vi "GetProperties.vi"(8 "error in":errorcluster, 11 "Boolean in":refnum<class "Boolean.lvclass">) -> (0 "error out":errorcluster, 3 "Boolean out":refnum<class "Boolean.lvclass">)   [LabVIEW 2014, in "Boolean.lvclass"]
uses:
  Boolean.lvclass
  Boolean.lvclass/Boolean.ctl
  Control/Control.lvclass
  Text/Text.lvclass
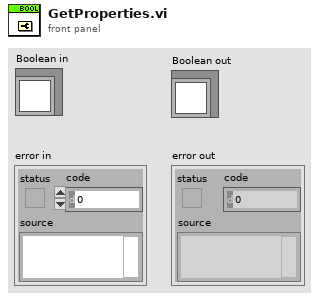
[diagram p1: front panel]
types:
  T1 = typedef "LVBoundsTypeDef.ctl" = cluster{"Width":u32, "Height":u32}
  T2 = typedef "LVKeyTypeDef.ctl" = cluster{"Focus":bool, "Control":bool, "Shift":bool, "Key":string}
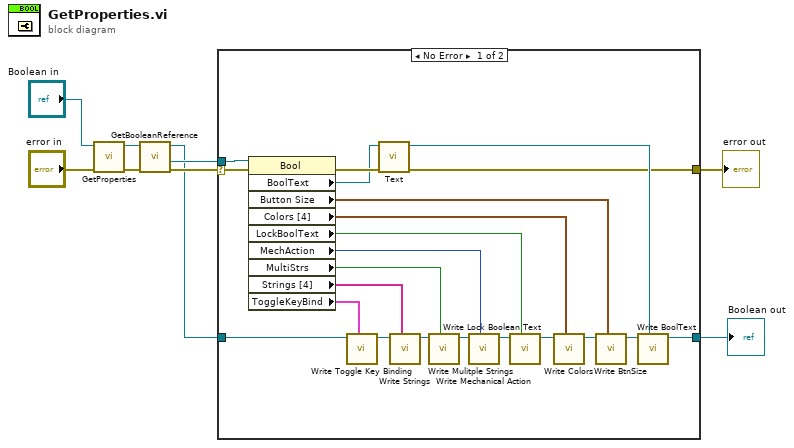
[diagram p0: block diagram]
diagram:
  n1 = call-parent "GetProperties.vi"("error in"="error in", "Control in"="Boolean in") -> ("error out"=w6:errorcluster, "Control out"=w7:refnum<class "Boolean.lvclass">)  [unwired: 8 in]
  n2 = call "GetBooleanReference.vi"("error in"=w6, "Boolean in"=w7) -> ("error out"=w5:errorcluster, "Boolean reference"=w4:refnum<vi>, "Boolean out"=w3:refnum<class "Boolean.lvclass">)  [unwired: 7 in]
  n3 = case shown="No Error" w5 {
    selector: w5 -> [w31 w32]
    tunnel: w4 -> [w30 _]
    tunnel: w3 -> [w12 w33]
    tunnel: [w11 w33] -> w1
    tunnel: [w10 w32] -> w2
    frame No Error {
      n4 = property class="Bool"(reference=w30, error in=w31) -> (error out=w29:errorcluster, "BoolText"=w28:refnum<vi>, "Button Size"=w24:T1, "Colors [4]"=w23:cluster{u32, u32}[], "LockBoolText"=w22:bool, "MechAction"=w19:u32, "MultiStrs"=w17:bool, "Strings [4]"=w15:string[], "ToggleKeyBind"=w13:T2)  [unwired: 1 out]
      n5 = call "Write Toggle Key Binding.vi"("Toggle Key Binding"=w13, "Boolean in"=w12) -> ("Boolean out"=w14:refnum<class "Boolean.lvclass">)  [unwired: 7 in]
      n6 = call "Text.vi"("error in"=w29, "GObj Refnum"=w28) -> ("error out"=w10:errorcluster, "Text out"=w25:refnum<class "Text.lvclass">)  [unwired: 8 in]
      n7 = call "Write Strings.vi"("Strings"=w15, "Boolean in"=w14) -> ("Boolean out"=w16:refnum<class "Boolean.lvclass">)  [unwired: 7 in]
      n8 = call "Write Mulitple Strings.vi"("Mulitple Strings"=w17, "Boolean in"=w16) -> ("Boolean out"=w18:refnum<class "Boolean.lvclass">)  [unwired: 7 in]
      n9 = call "Write Mechanical Action.vi"("Mechanical Action"=w19, "Boolean in"=w18) -> ("Boolean out"=w20:refnum<class "Boolean.lvclass">)  [unwired: 7 in]
      n10 = call "Write Lock Boolean Text.vi"("Lock Boolean Text"=w22, "Boolean in"=w20) -> ("Boolean out"=w21:refnum<class "Boolean.lvclass">)  [unwired: 7 in]
      n11 = call "Write Colors.vi"("Colors"=w23, "Boolean in"=w21) -> ("Boolean out"=w26:refnum<class "Boolean.lvclass">)  [unwired: 7 in]
      n12 = call "Write BtnSize.vi"("BtnSize"=w24, "Boolean in"=w26) -> ("Boolean out"=w27:refnum<class "Boolean.lvclass">)  [unwired: 7 in]
      n13 = call "Write BoolText.vi"("BoolText"=w25, "Boolean in"=w27) -> ("Boolean out"=w11:refnum<class "Boolean.lvclass">)  [unwired: 7 in]
    }
    frame Error {
    }
  }
  "error out" <- w2
  "Boolean out" <- w1
